vi "USRP Create AXI4-Lite Resources.vi"(0 "CLIP Resources\nFXP<+,32,32> Address\nFXP<+,32,32> Data":T1, 5 "UID for Dual Aurora x1 10.3125G CLIP":u16=1217) -> (4 "niInstr AXI4-Lite Address Space Collection v1 FPGA out":refnum<class "niInstr AXI4-Lite Address Space Collection v1 FPGA.lvclass">)   [LabVIEW 2016]
uses:
  <instrlib>/_niInstr/CLIP Adapters/v1/FPGA/AXI4-Lite/Address Space Collection/niInstr AXI4-Lite Address Space Collection v1 FPGA.lvclass
  <instrlib>/_niInstr/CLIP Adapters/v1/FPGA/AXI4-Lite/FXP32 Address - FXP32 Data/Public/CLIP Resources.ctl
  <instrlib>/_niInstr/Instruction Framework/v1/FPGA/Typedefs/Address Map Element.ctl
  <instrlib>/_niInstr/CLIP Adapters/v1/FPGA/AXI4-Lite/Address Space Collection/Private/Create Resources - FXP32 Address - FXP32 Data.vi
  <instrlib>/_niInstr/Instruction Framework/v1/FPGA/Typedefs/niInstr Instruction Framework v1 FPGA.lvlib
  <instrlib>/_niInstr/CLIP Adapters/v1/FPGA/AXI4-Lite/FXP32 Address - FXP32 Data/niInstr AXI4-Lite - FXP32 Address - FXP32 Data v1 FPGA.lvclass
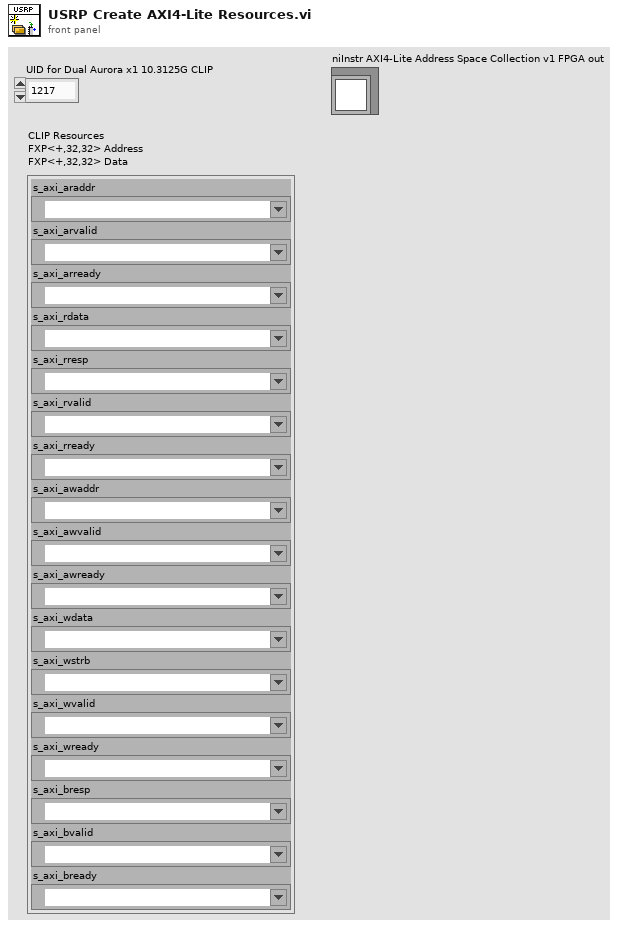
[diagram p1: front panel]
types:
  T1 = typedef "niInstr AXI4-Lite - FXP32 Address - FXP32 Data v1 FPGA.lvclass/CLIP Resources.ctl" = cluster{"s_axi_araddr":refnum<k21>, "s_axi_arvalid":refnum<k21>, "s_axi_arready":refnum<k21>, "s_axi_rdata":refnum<k21>, "s_axi_rresp":refnum<k21>, "s_axi_rvalid":refnum<k21>, "s_axi_rready":refnum<k21>, "s_axi_awaddr":refnum<k21>, "s_axi_awvalid":refnum<k21>, "s_axi_awready":refnum<k21>, "s_axi_wdata":refnum<k21>, "s_axi_wstrb":refnum<k21>, "s_axi_wvalid":refnum<k21>, "s_axi_wready":refnum<k21>, "s_axi_bresp":refnum<k21>, "s_axi_bvalid":refnum<k21>, "s_axi_bready":refnum<k21>}
  T2 = typedef "niInstr Instruction Framework v1 FPGA.lvlib/Address Map Element.ctl" = cluster{"UID":u16, "version":u16, "oldest compatible version":u16, "instance":u8, "number of children":u8, "offset":u32}
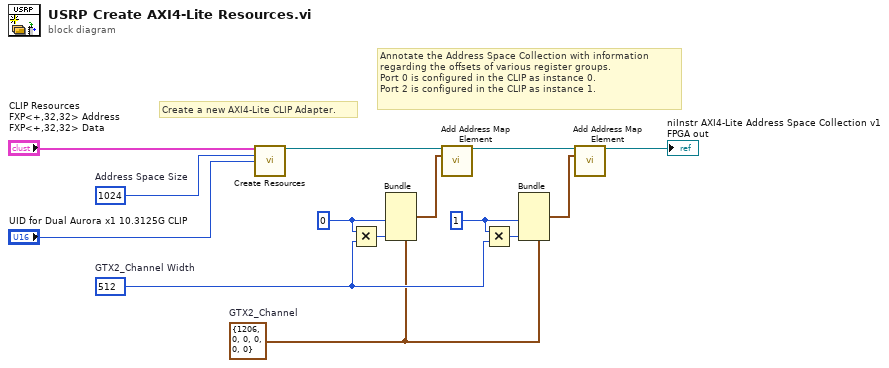
[diagram p0: block diagram]
diagram:
  w8 = u8 1 ("instance")
  w12 = T2 {"UID"=1206, "version"=0, "oldest compatible version"=0, "instance"=0, "number of children"=0, "offset"=0}  # GTX2_Channel
  w7 = u8 0 ("instance")
  w13 = u32 512  # GTX2_Channel Width
  w2 = u32 1024  # Address Space Size
  # "Annotate the Address Space Collection with information \nregarding the offsets of various register groups.\nPort 0 is configured in the CLIP as instance 0.\nPort 2 is configured in the CLIP as instance 1."
  # "Create a new AXI4-Lite CLIP Adapter."
  n1 = call-poly <instrlib>:"Create Resources.vi"("clip resources in"="CLIP Resources\nFXP<+,32,32> Address\nFXP<+,32,32> Data", "address space size"=w2, "address space uid"="UID for Dual Aurora x1 10.3125G CLIP") -> ("niInstr AXI4-Lite address space collection v1 FPGA out"=w4:refnum<class "niInstr AXI4-Lite Address Space Collection v1 FPGA.lvclass">)  [unwired: 12 in]
  n2 = Multiply(x=w7, y=w13) -> (x*y=w5:u32)
  n3 = Bundle(cluster=w12, "instance"=w7, "offset"=w5) -> (w6:T2)  [unwired: 4 in]
  n4 = call <instrlib>:"Add Address Map Element.vi"("niInstr AXI4-Lite address space collection v1 FPGA in"=w4, "address map element in"=w6) -> ("niInstr AXI4-Lite address space collection v1 FPGA out"=w10:refnum<class "niInstr AXI4-Lite Address Space Collection v1 FPGA.lvclass">)  [unwired: 13 in]
  n5 = Multiply(x=w8, y=w13) -> (x*y=w14:u32)
  n6 = Bundle(cluster=w12, "instance"=w8, "offset"=w14) -> (w9:T2)  [unwired: 4 in]
  n7 = call <instrlib>:"Add Address Map Element.vi"("niInstr AXI4-Lite address space collection v1 FPGA in"=w10, "address map element in"=w9) -> ("niInstr AXI4-Lite address space collection v1 FPGA out"=→"niInstr AXI4-Lite Address Space Collection v1 FPGA out":refnum<class "niInstr AXI4-Lite Address Space Collection v1 FPGA.lvclass">)  [unwired: 13 in]
